vi "MagSpecAnalyzeSingle.vi"(8 "error in (no error)":errorcluster, 10 "Image Src":T1, 11 "MagSpecCamera in":refnum<class "MagSpecCamera.lvclass">) -> (0 "error out":errorcluster, 1 "spectrum integrated in angle":T2, 2 "Iterpolated Image":dbl[][](graph), 3 "MagSpecCamera in 2":refnum<class "MagSpecCamera.lvclass">, 5 "time: 2Dinter":u32)   [LabVIEW 2020, in "MagSpecCamera.lvclass"]
uses:
  MagSpecCamera.lvclass
  IMAQ Image.ctl
  ScreenCam2_TypDEf.ctl
  CamAndObj_TypDEf.ctl
  MagSpecCamera.lvclass/MagSpecCamera.ctl
  NI_Vision_Development_Module.lvlib
panel:
  out "sum":dbl
  out "img 3":dbl[][](graph)
  out "img 2":u16[][](graph)
  out "img":dbl[][](graph)
  out "AngleAxis":dbl[](array[numeric])
  out "EnergyAxis":dbl[](array[numeric])
  out "Intensity Graph 2":u16[][](graph)
  out "charge >0.5":bool
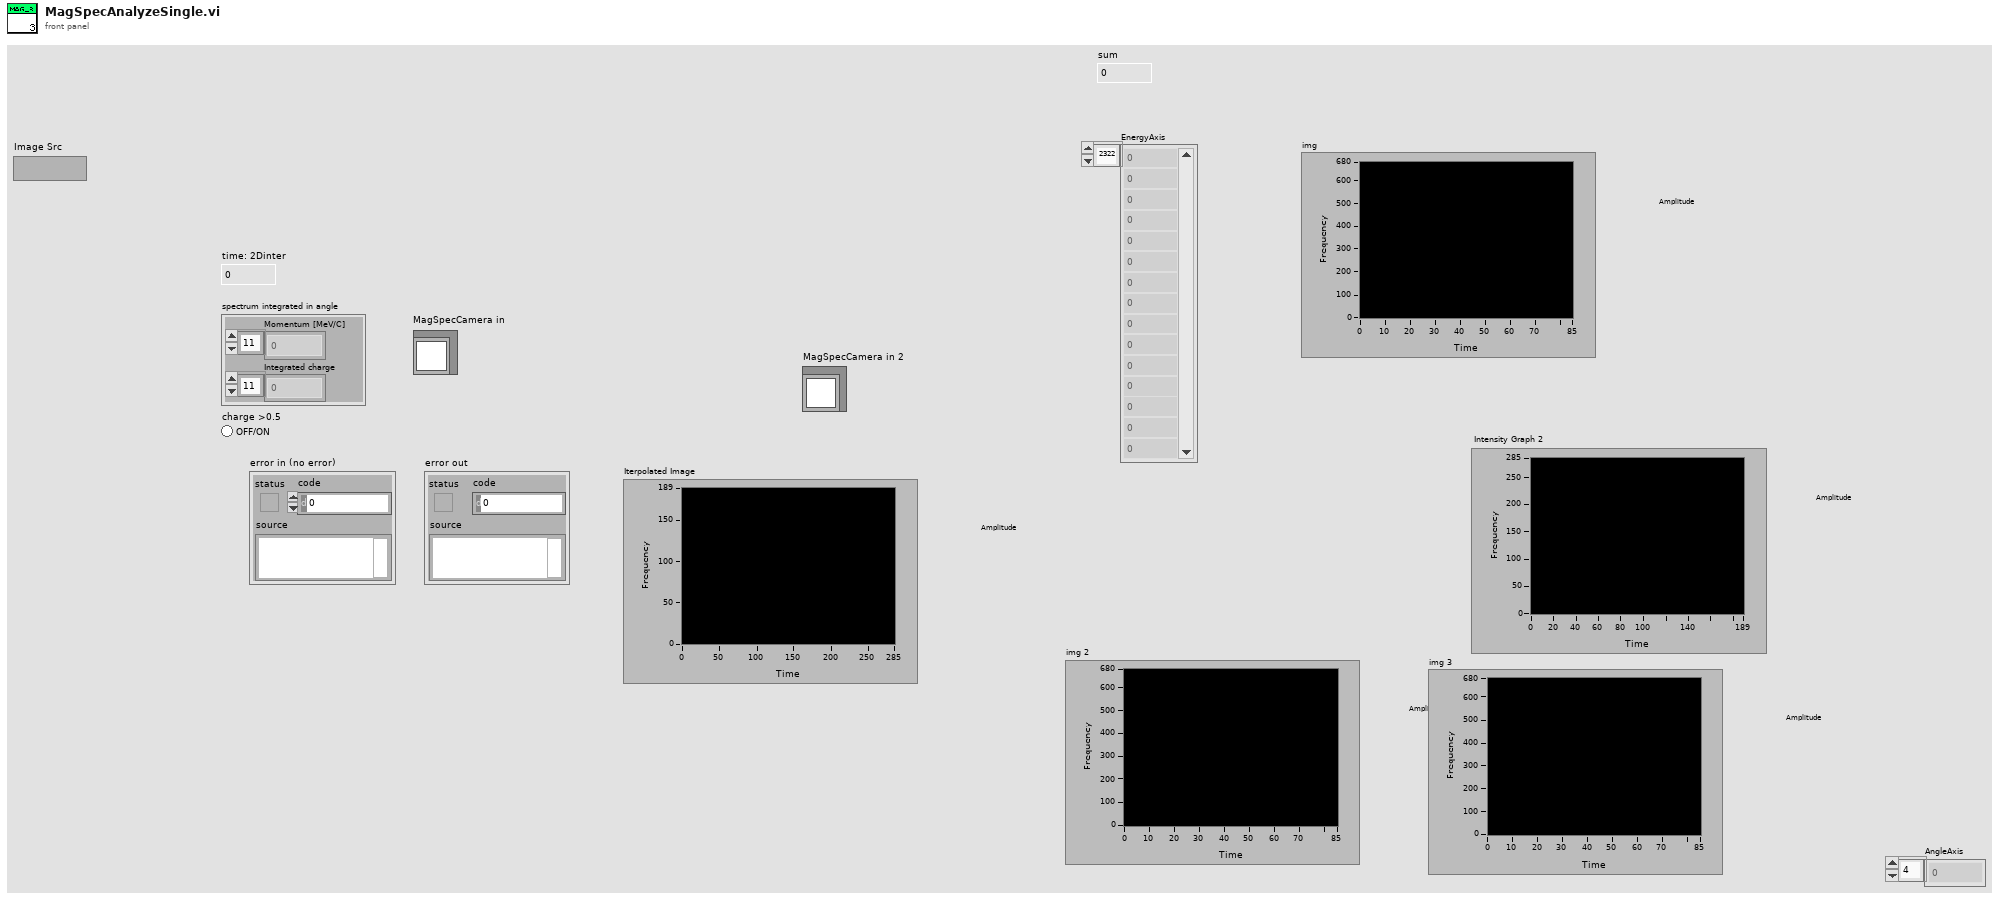
[diagram p1: front panel]
types:
  T1 = typedef "IMAQ Image.ctl" = refnum<image>
  T2 = cluster{"Momentum [MeV/C]":dbl[], "Integrated charge":dbl[]}
  T3 = cluster{"npix-X":i32, "npix-Y":i32, "Left [pix]":dbl, "Top [pix]":dbl}
  T4 = typedef "ScreenCam2_TypDEf.ctl" = cluster{"Screen Orientation":string, "Screen angle":string, "Lens":T5, "Calibration (mm/pix)":dbl}
  T5 = typedef "CamAndObj_TypDEf.ctl" = enum16{"FL1-f8x08", "FL1-f8x06", "FL1-f8", "ch300-f50", "FL2G-f8", "FL3M14-f8", "FL3M14-f8x08", "FL3M14-f8x08(2x2)", "aca720-f8", "aca1440-f8"}
  T6 = typedef "OnOffTypeDef.ctl" = enum16{"off", "on"}
  T7 = typedef "CameraSettings_File.ctl" = cluster{"FOV [mm]":dbl, "Left edge [mm]":dbl, "ROI Y offset":dbl, "ROI height":dbl, "ROI X offset":dbl, "ROI width":dbl, "Y center pixel":dbl, "Y Start":dbl, "Y End":dbl, "X Start":dbl, "X End":dbl, "rot [deg]":dbl}
  T8 = typedef "OneTimeCalculation.ctl" = cluster{"first Pixel pos [m]":dbl, "Pixel Size [mm]":dbl, "forward":T6}
  T9 = typedef "2D.ctl" = cluster{"dp":dbl[][], "chargeCompensation":dbl[][], "angle":dbl[][], "Momentum":dbl[][]}
  T10 = typedef "finalCalib--Cluster.ctl" = cluster{"X":dbl[][], "xi":dbl[][], "delta momentum":dbl, "Y":dbl[][], "yi":dbl[][], "angle (Y)":dbl[], "delta angle":dbl, "scale delta angle":dbl, "intraX":dbl, "intraY":dbl, "mask":dbl[][]}
  T11 = typedef "CamAndObj_TypDEf_Bella.ctl" = enum16{"FL1-f8x08", "FL1-f8x06", "FL1-f8", "ch300-f50", "FL2G-f8", "FL3M14-f8", "FL3M14-f8x08", "FL3M14-f8x08(2x2)", "aca720-f8", "aca1440-f8"}
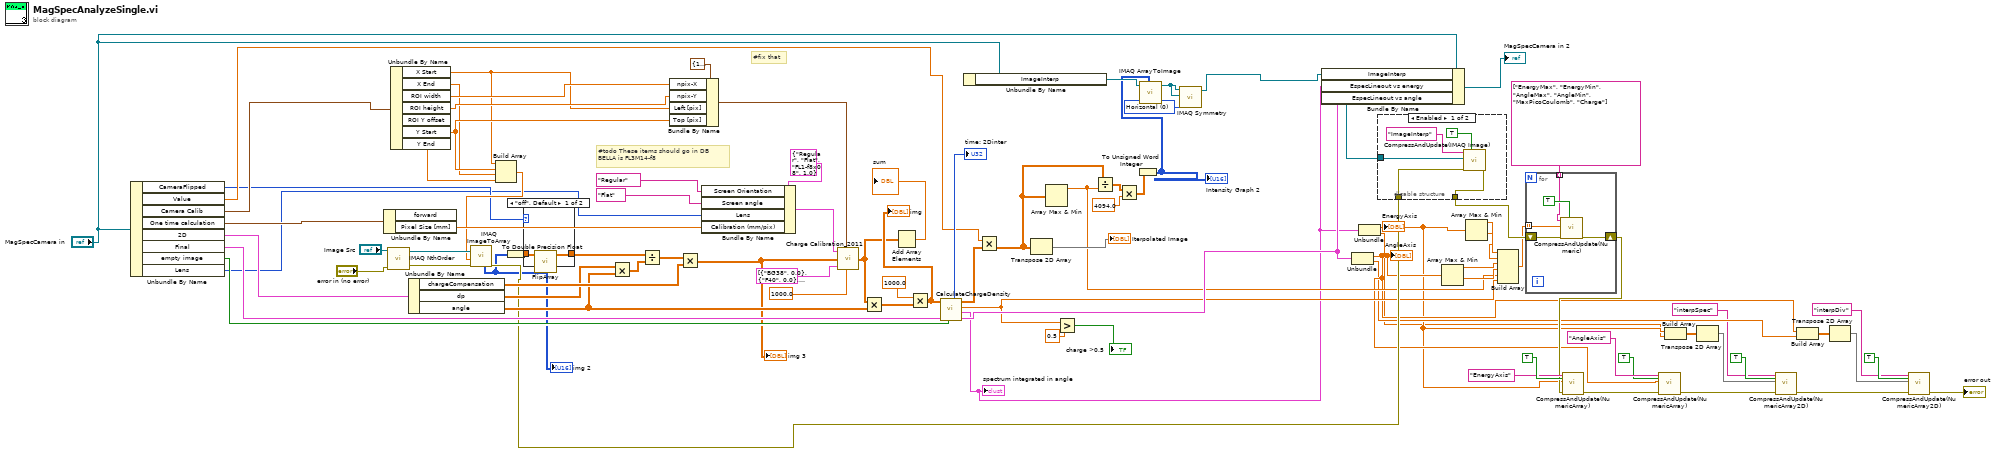
[diagram p0: block diagram]
diagram:
  w48 = u32 0 items=["Horizontal", "Vertical", "Central", "1st Diagonal", "2nd Diagonal"] ("Type of Symmetry")
  # "#fix that"
  # "#todo These items should go in DB\nBELLA is FL3M14-f8"
  n1 = Unbundle By Name("MagSpecCamera in") -> ("CameraFlipped"=w23:T6, "Value"=w39:dbl, "Camera Calib"=w63:T7, "One time calculation"=w62:T8, "2D"=w61:T9, "Final"=w60:T10, "empty image"=w59:bool, "Lens"=w19:T11)
  n2 = Unbundle By Name(w62) -> ("Pixel Size [mm]"=w65:dbl)  [unwired: 1 out]
  n3 = call "IMAQ NthOrder"("Image Src"="Image Src", "error in (no error)"="error in (no error)") -> ("Image Dst Out"=w83:T1, "error out"=w53:errorcluster)  [unwired: 5 in]
  n4 = Unbundle By Name(w63) -> ("X Start"=w79:dbl, "X End"=w74:dbl, "ROI width"=w81:dbl, "ROI height"=w82:dbl, "Y Start"=w80:dbl, "Y End"=w75:dbl)  [unwired: 1 out]
  n5 = Unbundle By Name(w61) -> ("chargeCompensation"=w73:dbl[][], "dp"=w72:dbl[][], "angle"=w64:dbl[][])
  n6 = Build Array(w79, w80, w74, w75) -> (w57:dbl[])
  n7 = call "IMAQ ImageToArray"("error in (no error)"=w53, "Optional Rectangle"=w57, "Image"=w83) -> ("Image Pixels (U16)"=w37:u16[][], "error out"=w51:errorcluster)  [unwired: 1 in, 3 out]
  "img 2" <- w37
  n8 = To Double Precision Float(number=w37) -> (double precision float=w77:dbl[][])
  n9 = case shown="\"off\", Default" w23 {
    tunnel: w77 -> [w93 w94]
    tunnel: [w92 w94] -> w78
    frame "off", Default {
      n10 = call "FlipArray.vi"("In"=w93) -> ("Out"=w92:dbl[][])  [unwired: 10 in]
    }
    frame "on" {
    }
  }
  n11 = Multiply(x=w72, y=w64) -> (x*y=w88:dbl[][])
  n12 = Divide(x=w78, y=w88) -> (x/y=w89:dbl[][])
  n13 = Bundle By Name(cluster=T3 {"npix-X"=1384, "npix-Y"=300, "Left [pix]"=0.0, "Top [pix]"=0.0} ("ROI infos"), "npix-X"=w81, "npix-Y"=w82, "Left [pix]"=w79, "Top [pix]"=w80) -> (w86:T3)
  n14 = Multiply(x=w89, y=w73) -> (x*y=w36:dbl[][])
  "img 3" <- w36
  n15 = Bundle By Name(cluster=T4 {"Screen Orientation"="Regular", "Screen angle"="Flat", "Lens"=enum."FL1-f8x08", "Calibration (mm/pix)"=1.0} ("Screen&Camera"), "Screen Orientation"="Regular", "Screen angle"="Flat", "Lens"=w19, "Calibration (mm/pix)"=w65) -> (w69:T4)
  n16 = call "Charge Calibration_2011.vi"("Screen&Camera 2"=w69, "ROI infos"=w86, "Image (Counts)"=w36, "Filters"=cluster{"Name":string, "#Filters":dbl}[] [{"Name"="BG38", "#Filters"=0.0}, {"Name"="F40", "#Filters"=0.0}, {"Name"="F70", "#Filters"=1.0}, {"Name"="oldBP", "#Filters"=0.0}], "Electron energy (MeV)"=1000.0) -> ("Image (pC)"=w18:dbl[][])  [unwired: 4 in]
  n17 = Multiply(x=w18, y=w64) -> (x*y=w84:dbl[][])
  n18 = Add Array Elements(numeric array=w18) -> (sum=→"sum":dbl)
  n19 = Multiply(x=1000.0, y=w84) -> (x*y=w38:dbl[][])
  "img" <- w38
  n20 = call "CalculateChargeDensity.vi"("empty image"=w59, "Final"=w60, "Z"=w38) -> ("Sum Y"=w47:cluster{"Ramp Pattern":dbl[], dbl[]}, "spec cluster 2"=w14:cluster{"Momentum [MeV/C]":dbl[], dbl[]}, "charge (sum)"=w22:dbl, "charge density"=w50:dbl[][], "time: 2Dinter"=→"time: 2Dinter":u32)  [unwired: 4 in]
  "spectrum integrated in angle" <- w14
  n21 = Unbundle By Name("MagSpecCamera in") -> ("ImageInterp"=w56:T1)
  n22 = Multiply(x=w39, y=w50) -> (x*y=w29:dbl[][])
  n23 = Transpose 2D Array(2D array=w29) -> (transposed array=→"Iterpolated Image":dbl[][])
  n24 = Array Max & Min(array=w29) -> (max value=w25:dbl)  [unwired: 3 out]
  n25 = Greater?(x=w22, y=0.5 ("change threshold")) -> (0:→"charge >0.5":bool)
  n26 = Divide(x=w29, y=w25) -> (x/y=w28:dbl[][])
  n27 = Multiply(x=w28, y=4094.0 ("max value")) -> (x*y=w26:dbl[][])
  n28 = To Unsigned Word Integer(number=w26) -> (unsigned 16bit integer=w55:u16[][])
  "Intensity Graph 2" <- w55
  n29 = call "IMAQ ArrayToImage"("Image Pixels (U16)"=w55, "Image"=w56) -> ("Image Out"=w21:T1)  [unwired: 8 in, 1 out]
  n30 = call "IMAQ Symmetry"("Type of Symmetry"=w48, "Image Dst"=w21, "Image Src"=w21) -> ("Image Dst Out"=w24:T1)  [unwired: 2 in, 1 out]
  n31 = Bundle By Name(cluster="MagSpecCamera in", "ImageInterp"=w24, "EspecLineout vs energy"=w14, "EspecLineout vs angle"=w47) -> (→"MagSpecCamera in 2":refnum<class "MagSpecCamera.lvclass">)
  n32 = Unbundle(w47) -> ("Ramp Pattern"=w16:dbl[], w15:dbl[])
  "AngleAxis" <- w16
  n33 = Unbundle(w14) -> ("Momentum [MeV/C]"=w7:dbl[], w6:dbl[])
  "EnergyAxis" <- w7
  n34 = disable-structure shown="Enabled" {
    disable-tunnel: w51 -> [w97 w100]
    disable-tunnel: w24 -> [w96 _]
    disable-tunnel: [w95 w100] -> w46
    frame Enabled {
      n35 = call "CompressAndUpdate(IMAQ Image).vi"("force CVT update (false)"=TRUE, "error in"=w97, "IMAQ Image"=w96, "command or variable name"="ImageInterp") -> ("error out"=w95:errorcluster)  [unwired: 7 in]
    }
    frame Disabled {
    }
  }
  n36 = Array Max & Min(array=w16) -> (max value=w42:dbl, min value=w41:dbl)  [unwired: 2 out]
  n37 = Array Max & Min(array=w7) -> (max value=w44:dbl, min value=w43:dbl)  [unwired: 2 out]
  n38 = Build Array(w44, w43, w42, w41, w25, w22) -> (w40:dbl[])
  n39 = for {
    shift-right: [w103] -> w31
    shift-left: w46 -> [w104]
    tunnel: string[] ["EnergyMax", "EnergyMin", "AngleMax", "AngleMin", "MaxPicoCoulomb", "Charge"] -> [w102] mode=indexing
    tunnel: w40 -> [w101] mode=indexing
    n40 = call "CompressAndUpdate(Numeric).vi"("force CVT update (false)"=TRUE, "error in"=w104, "Numeric"=w101, "command or variable name"=w102) -> ("error out"=w103:errorcluster)  [unwired: 7 in]
  }
  n41 = call "CompressAndUpdate(NumericArray).vi"("force CVT update (false)"=TRUE, "error in"=w31, "Numeric Array"=w7, "command or variable name"="EnergyAxis") -> ("error out"=w30:errorcluster)  [unwired: 7 in]
  n42 = call "CompressAndUpdate(NumericArray).vi"("force CVT update (false)"=TRUE, "error in"=w30, "Numeric Array"=w16, "command or variable name"="AngleAxis") -> ("error out"=w5:errorcluster)  [unwired: 7 in]
  n43 = Build Array(w7, w6) -> (w8:dbl[][])
  n44 = Transpose 2D Array(2D array=w8) -> (transposed array=w2:dbl[][])
  n45 = call "CompressAndUpdate(NumericArray2D).vi"("force CVT update (false)"=TRUE, "Error in"=w5, "Numeric Array 2D"=w2, "command or variable name"="interpSpec") -> ("Error out"=w4:errorcluster)  [unwired: 7 in]
  n46 = Build Array(w16, w15) -> (w10:dbl[][])
  n47 = Transpose 2D Array(2D array=w10) -> (transposed array=w9:dbl[][])
  n48 = call "CompressAndUpdate(NumericArray2D).vi"("force CVT update (false)"=TRUE, "Error in"=w4, "Numeric Array 2D"=w9, "command or variable name"="interpDiv") -> ("Error out"=→"error out":errorcluster)  [unwired: 7 in]
